vi "CreateSquare.vi"(6 "Color":u32(colorbox), 8 "Error In":errorcluster, 10 "a":dbl) -> (0 "Error Out":errorcluster, 3 "Square out":refnum<class "Square.lvclass">)   [LabVIEW 2021, in "Square.lvclass"]
doc: "Create a object of square class."
uses:
  Square.lvclass
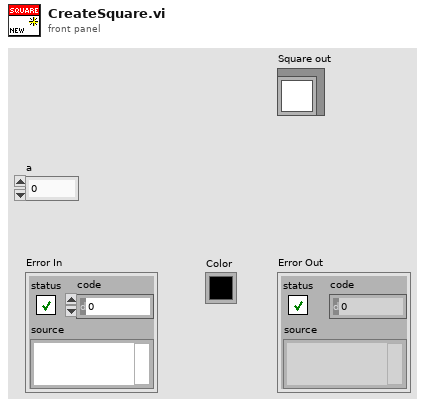
[diagram p1: front panel]
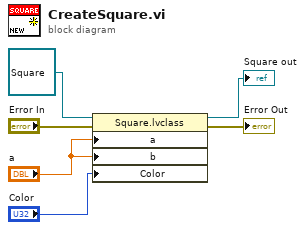
[diagram p0: block diagram]
diagram:
  n1 = property class="Square.lvclass"(reference=refnum<class "Square.lvclass"> refnum ("Square in"), error in="Error In", "a"="a", "b"="a", "Color"="Color") -> (reference out=→"Square out":refnum<class "Square.lvclass">, error out=→"Error Out":errorcluster)
